vi "signal_lim.vi"(1 "lim":dbl, 2 "x":dbl) -> (0 "y":dbl)   [LabVIEW 2019]
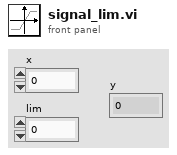
[diagram p1: front panel]
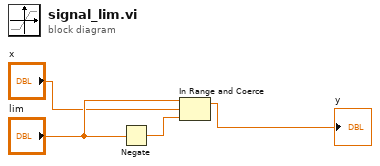
[diagram p0: block diagram]
diagram:
  n1 = Negate(x="lim") -> (-x=w4:dbl)
  n2 = In Range and Coerce(upper limit="lim", x="x", lower limit=w4) -> (coerced(x)=→"y":dbl)  [unwired: 1 out]
